vi "Increment_Time_Auto.vi"(10 "Value":T1(array[cluster])) -> (3 "Array":T1(array[cluster]))   [LabVIEW 2013]
doc: "Upon Clean Up:\n Increments time in Timing Sequence or Timing Sequence 2 (input property node) for those set to 'Auto'"
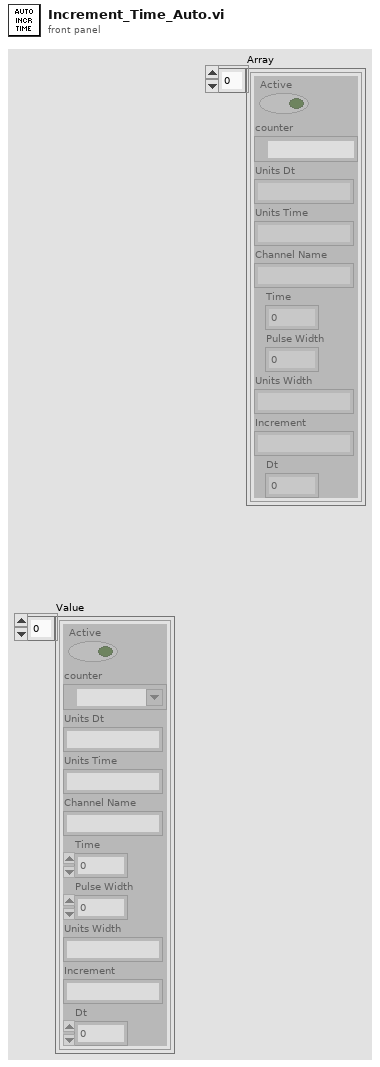
[diagram p1: front panel]
types:
  T1 = cluster{"Active":bool, "counter":tag, "Units Dt":string, "Units Time":string, "Channel Name":string, "Time":dbl, "Pulse Width":dbl, "Units Width":string, "Increment":string, "Dt":dbl}[]
  T2 = cluster{"Active":bool, "counter":tag, "Units Dt":string, "Units Time":string, "Channel Name":string, "Time":dbl, "Pulse Width":dbl, "Units Width":string, "Increment":string, "Dt":dbl}
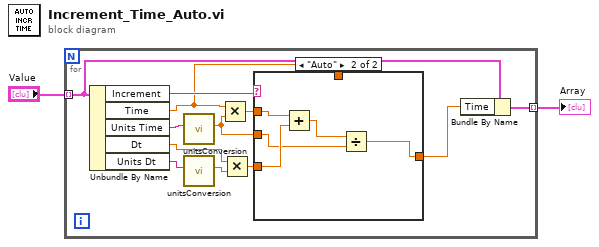
[diagram p0: block diagram]
diagram:
  n1 = for {
    tunnel: "Value" -> [w7] mode=indexing
    tunnel: [w13] -> w2 mode=indexing
    n2 = Unbundle By Name(w7) -> ("Increment"=w14:string, "Time"=w8:dbl, "Units Time"=w6:string, "Dt"=w12:dbl, "Units Dt"=w4:string)
    n3 = call "unitsConversion.vi"("Units"=w6) -> ("Numeric"=w5:dbl)  [unwired: 10 in]
    n4 = call "unitsConversion.vi"("Units"=w4) -> ("Numeric"=w3:dbl)  [unwired: 10 in]
    n5 = Multiply(x=w8, y=w5) -> (x*y=w11:dbl)
    n6 = Multiply(x=w12, y=w3) -> (x*y=w10:dbl)
    n7 = case shown="\"Auto\"" w14 {
      tunnel: w11 -> [_ w20]
      tunnel: w10 -> [_ w19]
      tunnel: w5 -> [_ w17]
      tunnel: [w15 w16] -> w9
      tunnel: w8 -> [w15 _]
      frame "False", Default {
      }
      frame "Auto" {
        n8 = Add(x=w20, y=w19) -> (x+y=w18:dbl)
        n9 = Divide(x=w18, y=w17) -> (x/y=w16:dbl)
      }
    }
    n10 = Bundle By Name(cluster=w7, "Time"=w9) -> (w13:T2)
  }
  "Array" <- w2
